vi "Subvi SetFileName.vi"(1 "Thickness":u16, 2 "SectionNumInFile":u32 max=10000, 3 "BaseFile":string) -> (0 "ImageFile":string)   [LabVIEW 2012]
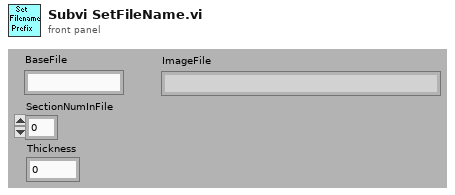
[diagram p1: front panel]
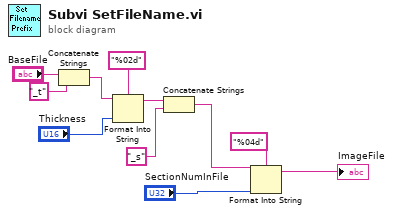
[diagram p0: block diagram]
diagram:
  n1 = Concatenate Strings("BaseFile", "_t" ("string")) -> (w8:string)
  n2 = Format Into String(format string="%02d", initial string=w8, "Thickness") -> (resulting string=w6:string)  [unwired: 1 in, 1 out]
  n3 = Concatenate Strings(w6, "_s" ("format string")) -> (w3:string)
  n4 = Format Into String(format string="%04d", initial string=w3, "SectionNumInFile") -> (resulting string=→"ImageFile":string)  [unwired: 1 in, 1 out]
